vi "Tray_TrayInitial.vi"(6 "Initial color":u32(colorbox)=16860, 8 "error in (no error)":errorcluster, 9 "SetColor":bool, 10 "TrayCase":i32, 11 "TrayIn":refnum<vi>) -> (0 "error Out":errorcluster)   [LabVIEW 2019]
uses:
  global/Tray_ArrAndData.vi
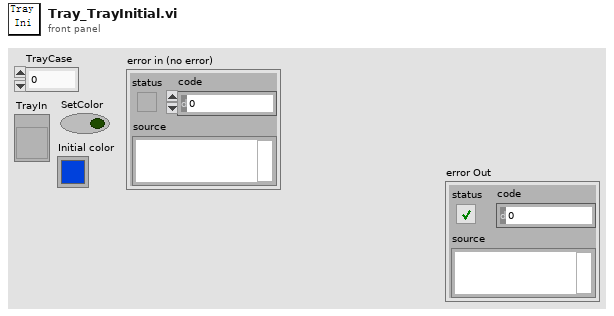
[diagram p1: front panel]
types:
  T1 = cluster{"XY_ATray":cluster{"X":i32, "Y":i32}, "Initial color":u32, "FinalColor":u32}
  T2 = cluster{"XY_BTray":cluster{"X":i32, "Y":i32}, "Initial color":u32, "FinalColor":u32}
  T3 = cluster{"XY_CTray":cluster{"X":i32, "Y":i32}, "Initial color":u32, "FinalColor":u32}
  T4 = cluster{"XY_DTray":cluster{"X":i32, "Y":i32}, "Initial color":u32, "FinalColor":u32}
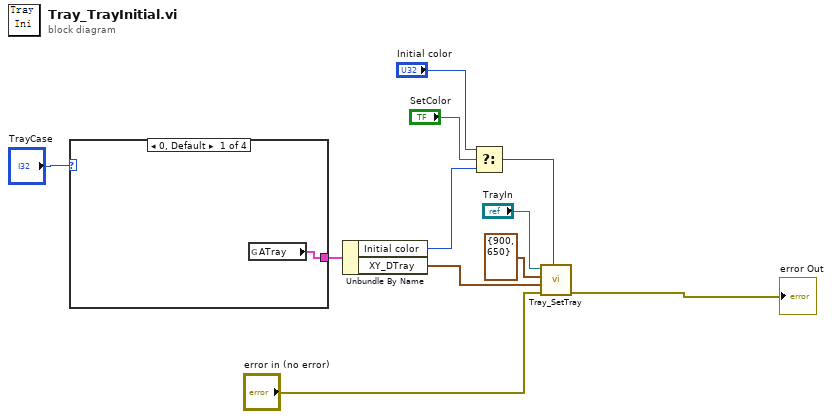
[diagram p0: block diagram]
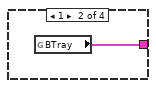
[diagram p2: hidden frame]
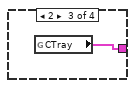
[diagram p3: hidden frame]
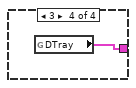
[diagram p4: hidden frame]
diagram:
  n1 = case shown="0, Default" "TrayCase" {
    tunnel: [w12 w13 w14 w15] -> w3
    frame 0, Default {
      n2 = global read "Tray_ArrAndData.vi" "ATray"() -> (w12:T1)
    }
    frame 1 {
      n3 = global read "Tray_ArrAndData.vi" "BTray"() -> (w13:T2)
    }
    frame 2 {
      n4 = global read "Tray_ArrAndData.vi" "CTray"() -> (w14:T3)
    }
    frame 3 {
      n5 = global read "Tray_ArrAndData.vi" "DTray"() -> (w15:T4)
    }
  }
  n6 = Unbundle By Name(w3) -> ("Initial color"=w2:u32, "XY_DTray"=w1:cluster{"X":i32, "Y":i32})
  n7 = Select(t="Initial color", s="SetColor", f=w2) -> (s? t:f=w6:u32)
  n8 = call "Tray_SetTray.vi"("Initial color"=w6, "error in (no error)"="error in (no error)", "GridSize"=w1, "MaxArea"=cluster{"x":u32, "y":u32} {"x"=900, "y"=650}, "Tray in"="TrayIn") -> ("error out"=→"error Out":errorcluster)  [unwired: 6 in]
